vi "initial_mkdir.vi"(8 "error in":errorcluster) -> (0 "error out":errorcluster)   [LabVIEW 2024]
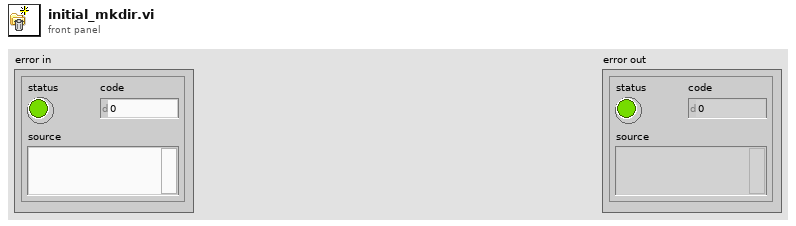
[diagram p1: front panel]
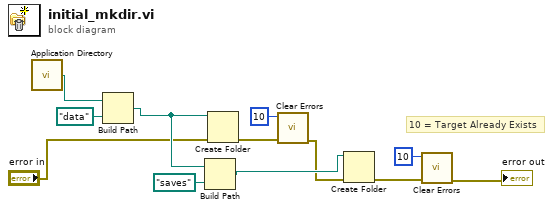
[diagram p0: block diagram]
diagram:
  # "10 = Target Already Exists"
  n1 = call <vilib>:"Application Directory.vi"() -> ("Application Directory"=w12:path)
  n2 = Build Path(base path=w12, name or relative path=path "data") -> (appended path=w9:path)
  n3 = Build Path(base path=w9, name or relative path=path "saves") -> (appended path=w10:path)
  n4 = Create Folder(path (use dialog)=w9, error in="error in") -> (error out=w2:errorcluster)  [unwired: 1 in, 2 out]
  n5 = call <vilib>:"Clear Errors.vi"("error in (no error)"=w2, "specific error code to clear (0: all)"=10) -> ("error out"=w1:errorcluster)  [unwired: 4 in, 1 out]
  n6 = Create Folder(path (use dialog)=w10, error in=w1) -> (error out=w6:errorcluster)  [unwired: 1 in, 2 out]
  n7 = call <vilib>:"Clear Errors.vi"("error in (no error)"=w6, "specific error code to clear (0: all)"=10) -> ("error out"=→"error out":errorcluster)  [unwired: 4 in, 1 out]
